vi "CS-Aperture size display.vi"(6 "实际孔径":dbl, 8 "error in (no error)":errorcluster caption="错误输入（无错误）", 9 "孔径规格":T2, 10 "ROI Descriptor":T3 {"Contours"."Type" items=["No Selection", "Point", "Line", "Rectangle", "Oval", "Polygon", "Freehand Region", "Annulus", "Unused2", "Unused3", "Broken Line", "Freehand Line", "Rotated Rectangle"]}, 11 "原始图像 IN":T4(plugin-control)) -> (0 "error out":errorcluster caption="错误输出", 2 "结果":string[](array[string]), 3 "原始图像 OUT":T4(plugin-control), 4 "异常":bool, 5 "OK/NG":bool)   [LabVIEW 2017]
panel:
  out "String 2":string="NG"
  out "String":string="OK"
  in  "Bounding Rectangle":T1
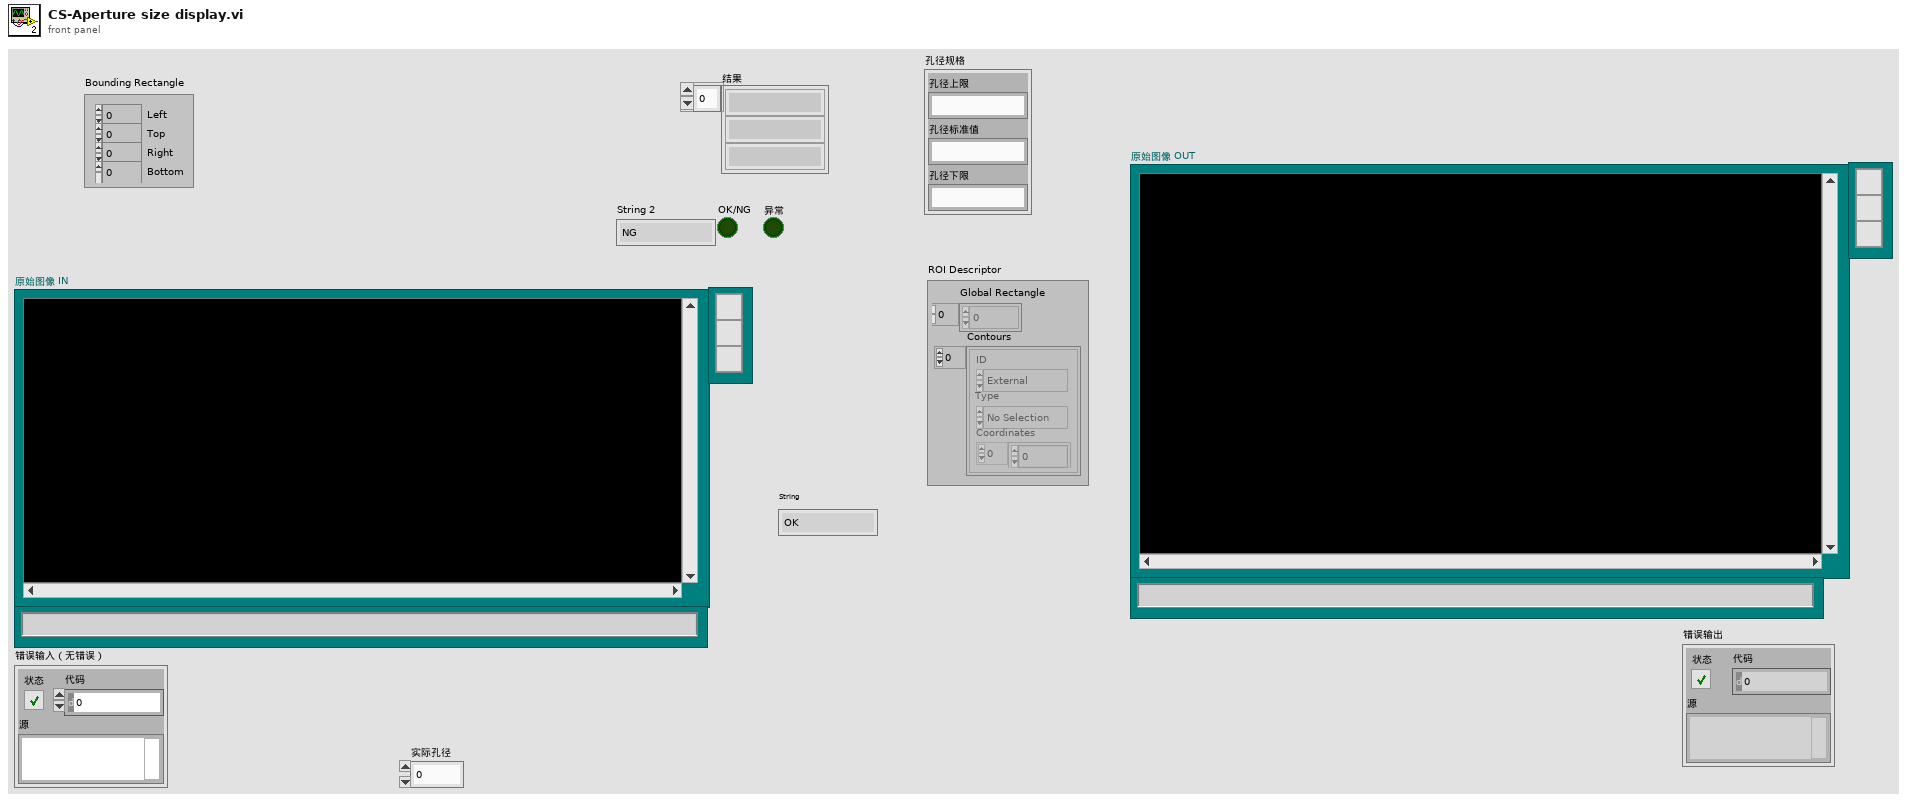
[diagram p1: front panel]
types:
  T1 = cluster{"Left":i32, "Top":i32, "Right":i32, "Bottom":i32}
  T2 = cluster{"孔径上限":string, "孔径标准值":string, "孔径下限":string}
  T3 = typedef "ROI Descriptor" = cluster{"Global Rectangle":i32[], "Contours":cluster{"ID":enum32{"External", "Internal"}, "Type":u32, "Coordinates":i32[]}[]}
  T4 = typedef "IMAQ Image.ctl" = refnum<image>
  T5 = cluster{"Desired Font (Application)":enum16{"User-specified Font", "Application Font", "System Font", "Dialog Font"}, "[User-specified Font]":cluster{"Font Name":string, "Size":i16, "Strikeout?":bool, "Italic?":bool, "Underline?":bool, "Outline?":bool, "Shadow?":bool, "Bold?":bool, "Rotation Angle":dbl}, "Horizontal Alignment":i16, "Vertical Alignment":i16}
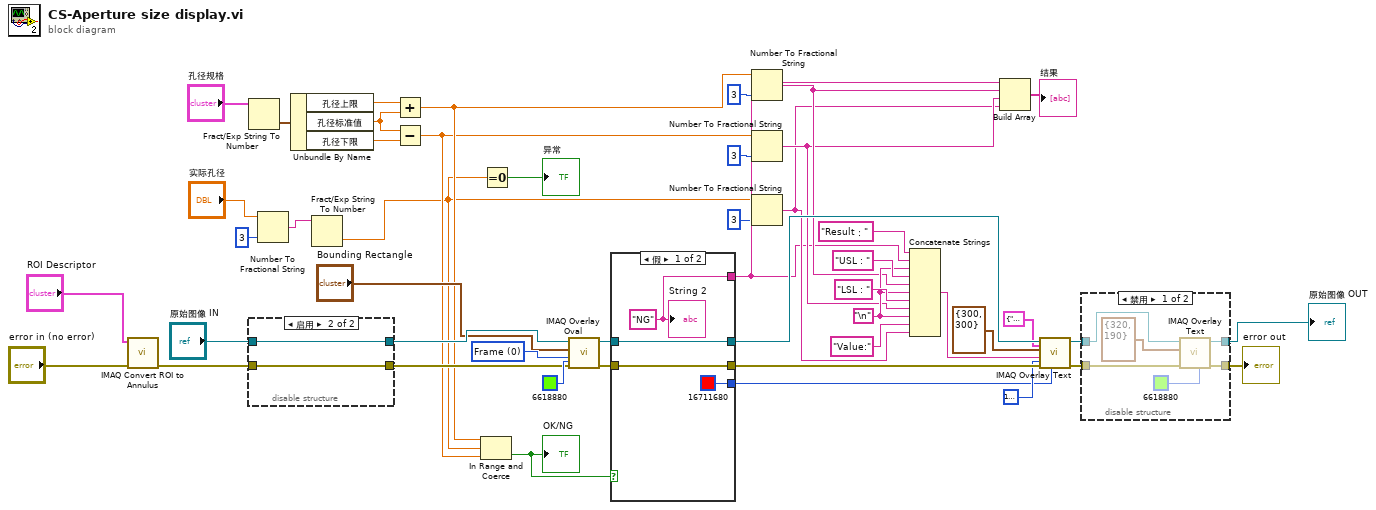
[diagram p0: block diagram]
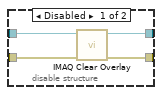
[diagram p2: hidden frame]
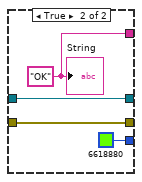
[diagram p4: hidden frame]
diagram:
  w12 = "\n"
  w28 = u32 0 items=["Frame", "Fill"] ("Drawing Mode (Frame)")
  n1 = call "IMAQ Convert ROI to Annulus"("error in (no error)"="error in (no error)", "ROI Descriptor"="ROI Descriptor") -> ("error out"=w37:errorcluster)  [unwired: 7 in, 1 out]
  n2 = Fract/Exp String To Number(string="孔径规格") -> (number=w32:cluster{"孔径上限":dbl, "孔径标准值":dbl, "孔径下限":dbl})  [unwired: 3 in, 1 out]
  n3 = disable-structure shown="启用" {
    disable-tunnel: "原始图像 IN" -> [w52 w54]
    disable-tunnel: [w51 w54] -> w38
    disable-tunnel: w37 -> [w50 w53]
    disable-tunnel: [w49 w53] -> w36
    frame Disabled {
      n4 = call "IMAQ Clear Overlay"("error in (no error)"=w50, "Image"=w52) -> ("error out"=w49:errorcluster, "Image Out"=w51:T4)  [unwired: 8 in]
    }
    frame Enabled {
    }
  }
  n5 = Number To Fractional String(number="实际孔径", precision (6)=i16 3 ("精度(6)")) -> (F-format string=w4:string)  [unwired: 2 in]
  n6 = Unbundle By Name(w32) -> ("孔径上限"=w31:dbl, "孔径标准值"=w30:dbl, "孔径下限"=w29:dbl)
  n7 = Fract/Exp String To Number(string=w4) -> (number=w2:dbl)  [unwired: 3 in, 1 out]
  n8 = Add(x=w31, y=w30) -> (x+y=w20:dbl)
  n9 = Subtract(x=w30, y=w29) -> (x-y=w17:dbl)
  n10 = In Range and Coerce(upper limit=w20, x=w2, lower limit=w17) -> (In Range?=w21:bool)  [unwired: 1 out]
  "OK/NG" <- w21
  n11 = Equal To 0?(x=w2) -> (x = 0?=→"异常":bool)
  n12 = call "IMAQ Overlay Oval"("Color"=u32 6618880, "error in (no error)"=w36, "Drawing Mode (Frame)"=w28, "Bounding Rectangle"="Bounding Rectangle", "Image"=w38) -> ("error out"=w34:errorcluster, "Image Out"=w35:T4)  [unwired: 5 in]
  n13 = case shown="假" w21 {
    tunnel: w35 -> [w58 w62]
    tunnel: w34 -> [w57 w61]
    tunnel: [w58 w62] -> w44
    tunnel: [w57 w61] -> w43
    tunnel: [w56 w59] -> w6
    tunnel: [u32 16711680 ("Text Color (black)") u32 6618880 ("Text Color (black)")] -> w40
    frame False {
      w56 = "NG" ("String")
      "String 2" <- w56
    }
    frame True {
      w59 = "OK" ("String")
      "String" <- w59
    }
  }
  n14 = Number To Fractional String(number=w20, precision (6)=i16 3 ("精度(6)")) -> (F-format string=w10:string)  [unwired: 2 in]
  n15 = Number To Fractional String(number=w17, precision (6)=i16 3 ("精度(6)")) -> (F-format string=w9:string)  [unwired: 2 in]
  n16 = Number To Fractional String(number=w2, precision (6)=i16 3 ("精度(6)")) -> (F-format string=w7:string)  [unwired: 2 in]
  n17 = Concatenate Strings("Result：" ("字符串"), w6, w12, "USL : " ("字符串"), w10, w12, "LSL : " ("字符串"), w9, w12, "Value:" ("字符串"), w7) -> (w14:string)
  n18 = Build Array(w6, w10, w9, w7) -> (→"结果":string[])
  n19 = call "IMAQ Overlay Text"("BG Color (Transparent)"=u32 16777216, "Text Color (black)"=w40, "Font, Size & Style"=T5 {"Desired Font (Application)"=enum."User-specified Font", "[User-specified Font]"={"Font Name"="", "Size"=100, "Strikeout?"=FALSE, "Italic?"=FALSE, "Underline?"=FALSE, "Outline?"=FALSE, "Shadow?"=FALSE, "Bold?"=TRUE, "Rotation Angle"=0.0}, "Horizontal Alignment"=0, "Vertical Alignment"=0}, "error in (no error)"=w43, "String"=w14, "Origin"=cluster{"X":i32, "Y":i32} {"X"=300, "Y"=300}, "Image"=w44) -> ("error out"=w24:errorcluster, "Image Out"=w26:T4)  [unwired: 3 in]
  n20 = disable-structure shown="禁用" {
    disable-tunnel: w26 -> [w68 w70]
    disable-tunnel: [w67 w70] -> w25
    disable-tunnel: w24 -> [w66 w69]
    disable-tunnel: [w65 w69] -> w23
    frame Disabled {
      n21 = call "IMAQ Overlay Text"("BG Color (Transparent)"=u32 6618880, "error in (no error)"=w66, "Origin"=cluster{"X":i32, "Y":i32} {"X"=320, "Y"=190}, "Image"=w68) -> ("error out"=w65:errorcluster, "Image Out"=w67:T4)  [unwired: 6 in]
    }
    frame Enabled {
    }
  }
  "原始图像 OUT" <- w25
  "error out" <- w23
